vi "GetQueues.vi"(11 "create new? (F)":bool) -> (1 "User Interface Camera Control":refnum<queue>, 3 "Queue List":T1)   [LabVIEW 2011]
uses:
  Typedefs/QueueListType.ctl
  Typedefs/Cmd_MotorIn.ctl
  Typedefs/CmdEnum_MotorIn.ctl
  Typedefs/CmdData_NewFrame.ctl
  <vilib>/vision/Image Controls.llb/IMAQ Image.ctl
  Typedefs/CmdEnum_CameraFrameType.ctl
  Typedefs/UserInterfaceEventType.ctl
  Typedefs/CmdEnum_UserInterfaceCmd.ctl
  GlobalVariables.vi
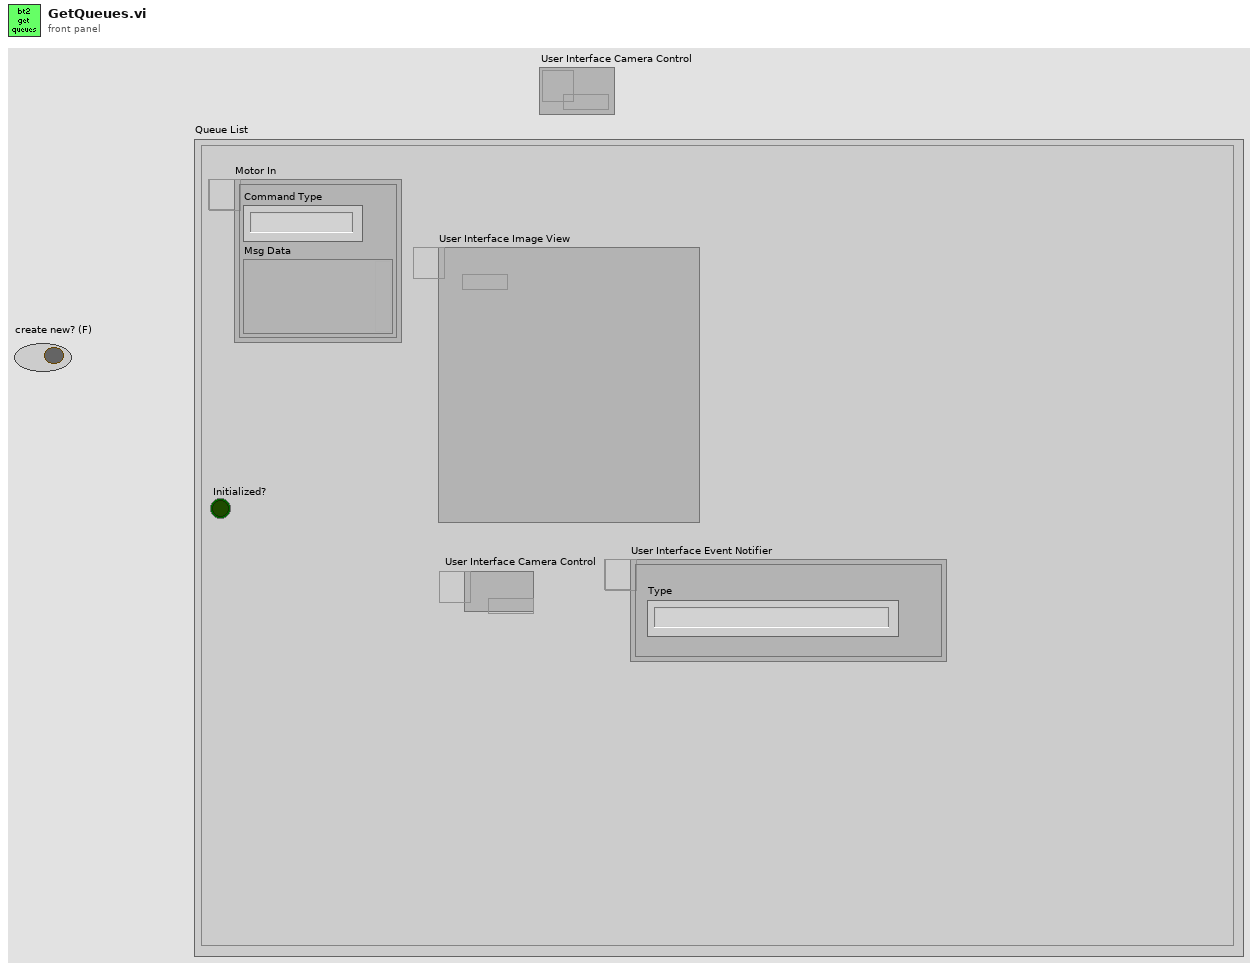
[diagram p1: front panel]
types:
  T1 = typedef "QueueListType.ctl" = cluster{"Motor In":refnum<queue>, "User Interface Image View":refnum<queue>, "User Interface Camera Control":refnum<queue>, "User Interface Event Notifier":refnum<notifier>, "Initialized?":bool}
  T2 = typedef "UserInterfaceEventType.ctl" = cluster{"Type":T3}
  T3 = typedef "CmdEnum_UserInterfaceCmd.ctl" = enum32{"Idle (Use for default)", "ResultTracesUpdated", "MeasureConfigUpdated", "MeasureEnd", "MeasureStart"}
  T4 = typedef "Cmd_MotorIn.ctl" = cluster{"Command Type":T5, "Msg Data":variant}
  T5 = typedef "CmdEnum_MotorIn.ctl" = enum32{"Init", "Close", "SetPosition", "UpdatePositions", "MoveToLimit"}
  T6 = typedef "CmdData_NewFrame.ctl" = cluster{"Buffer Image":T7, "Frame #":i32, "Hardware ROI Index":i32, "Timestamp":dbl, "Type":T8}
  T7 = typedef "IMAQ Image.ctl" = refnum<image>
  T8 = typedef "CmdEnum_CameraFrameType.ctl" = enum16{"Full", "HardwareROI", "EndGrabMarker"}
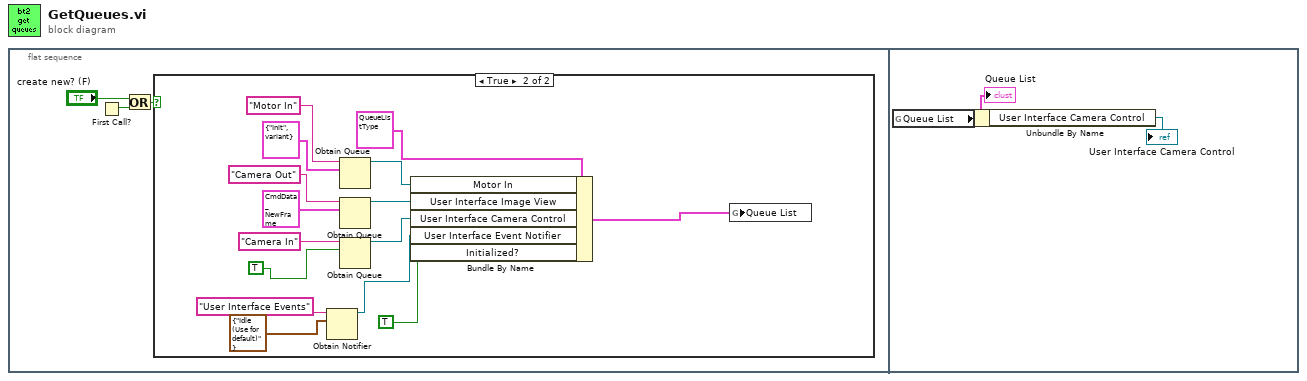
[diagram p0: block diagram]
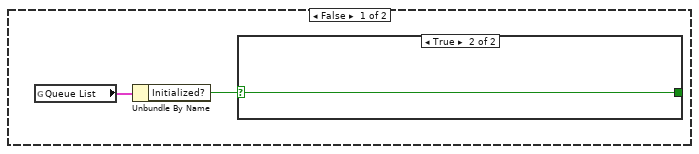
[diagram p2: hidden frame]
diagram:
  n1 = flat-sequence {
    frame #0 {
      n2 = First Call?() -> (First Call?: T/F=w3:bool)
      n3 = Or(x="create new? (F)", y=w3) -> (x .or. y?=w1:bool)
      n4 = case shown="True" w1 {
        frame False {
          n5 = global read "GlobalVariables.vi" "Queue List"() -> (w5:T1)
          n6 = Unbundle By Name(w5) -> ("Initialized?"=w4:bool)
          n7 = case shown="True" w4 {
            selector: w4 -> [w6 w7]
            tunnel: [w6 w7] -> _
            frame False {
              # "If you hit this breakpoint, you are not starting \nthe program through MainUI.vi"
            }
            frame True {
            }
          }
        }
        frame True {
          n8 = Obtain Notifier(name (unnamed)="User Interface Events", notification data type=T2 {"Type"=enum."Idle (Use for default)"} ("User Interface Event")) -> (notifier out=w9:refnum<notifier>)  [unwired: 2 in, 2 out]
          n9 = Obtain Queue(name (unnamed)="Motor In", element data type=T4 {"Command Type"=enum."Init", "Msg Data"=variant}) -> (queue out=w16:refnum<queue>)  [unwired: 3 in, 2 out]
          n10 = Obtain Queue(name (unnamed)="Camera Out", element data type=T6 {"Buffer Image"=refnum, "Frame #"=0, "Hardware ROI Index"=0, "Timestamp"=0.0, "Type"=enum."Full"} ("Cluster")) -> (queue out=w12:refnum<queue>)  [unwired: 3 in, 2 out]
          n11 = Obtain Queue(name (unnamed)="Camera In", element data type=TRUE) -> (queue out=w15:refnum<queue>)  [unwired: 3 in, 2 out]
          n12 = Bundle By Name(cluster=T1 {"Motor In"=refnum, "User Interface Image View"=refnum, "User Interface Camera Control"=refnum, "User Interface Event Notifier"=refnum, "Initialized?"=FALSE} ("Queue List"), "Motor In"=w16, "User Interface Image View"=w12, "User Interface Camera Control"=w15, "User Interface Event Notifier"=w9, "Initialized?"=TRUE) -> (w13:T1)
          n13 = global write "GlobalVariables.vi" "Queue List"(w13) -> ()
        }
      }
    }
    frame #1 {
      n14 = global read "GlobalVariables.vi" "Queue List"() -> (w24:T1)
      "Queue List" <- w24
      n15 = Unbundle By Name(w24) -> ("User Interface Camera Control"=→"User Interface Camera Control":refnum<queue>)
    }
  }
